vi "EOLmarkerGenerator.vi"(8 "chunk":i16[](array[numeric]), 9 "Polarity":bool, 10 "markerValue":i16=10000, 11 "markerArrayIn":i16[](array[numeric])) -> (3 "markerArrayOut":i16[](array[numeric]))   [LabVIEW 2022 SP3]
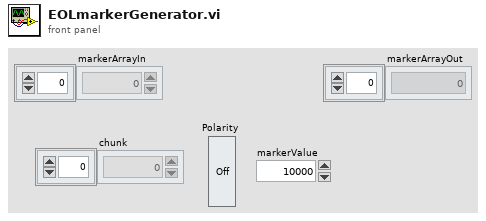
[diagram p1: front panel]
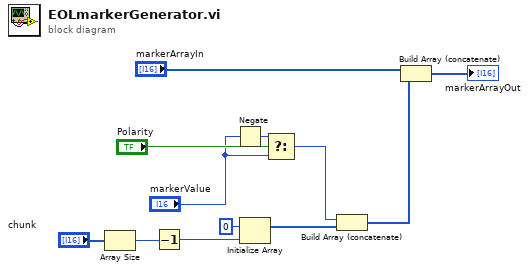
[diagram p0: block diagram]
diagram:
  n1 = Array Size(array="chunk") -> (size(s)=w11:i32)
  n2 = Decrement(x=w11) -> (x-1=w8:i32)
  n3 = Negate(x="markerValue") -> (-x=w6:i16)
  n4 = Initialize Array(i16 0, w8) -> (w10:i16[])
  n5 = Select(t=w6, s="Polarity", f="markerValue") -> (s? t:f=w4:i16)
  n6 = Build Array (concatenate)(w4, w10) -> (w2:i16[])
  n7 = Build Array (concatenate)("markerArrayIn", w2) -> (→"markerArrayOut":i16[])
